vi "Problema3_2.vi"() -> ()   [LabVIEW 2020]
panel:
  out "Valor final del coseno":dbl
  out "Maximo":dbl[](array[numeric])
  out "?":dbl[][](graph)
  # "Señales de las funciones Seno y Coseno."
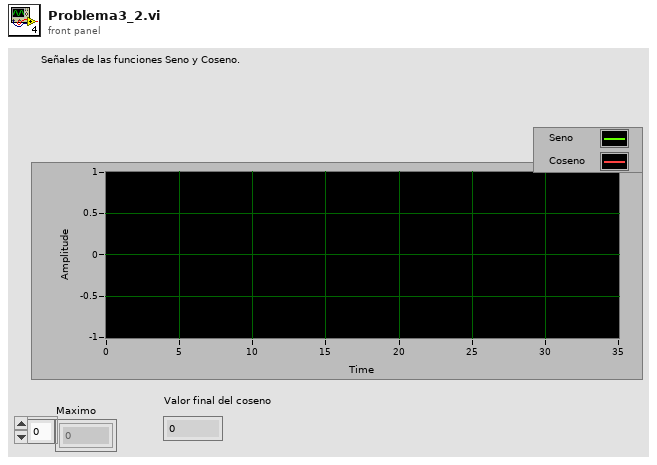
[diagram p1: front panel]
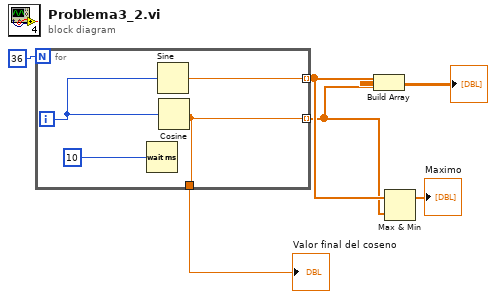
[diagram p0: block diagram]
diagram:
  n1 = for {
    N: 36 -> [_]
    tunnel: [w10] -> w4 mode=indexing
    tunnel: [w7] -> w3 mode=indexing
    tunnel: [w7] -> w1
    i -> [w8]
    n2 = Wait (ms)(milliseconds to wait=u32 10) -> ()  [unwired: 1 out]
    n3 = Sine(x=w8) -> (sin(x)=w10:dbl)
    n4 = Cosine(x=w8) -> (cos(x)=w7:dbl)
  }
  "Valor final del coseno" <- w1
  n5 = Build Array(w4, w3) -> (→"?":dbl[][])
  n6 = Max & Min(x=w4, y=w3) -> (max(x,y)=→"Maximo":dbl[])  [unwired: 1 out]
